vi "实验1-1.vi"() -> ()   [LabVIEW 2018]
panel:
  out "a*10":dbl
  out "?":bool
  in  "b":dbl
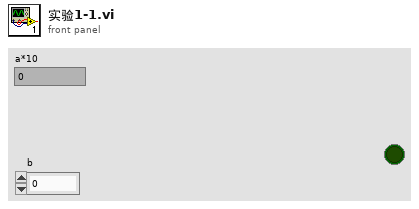
[diagram p1: front panel]
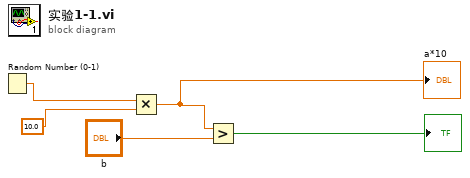
[diagram p0: block diagram]
diagram:
  n1 = Random Number (0-1)() -> (number: 0 to 1=w4:dbl)
  n2 = Multiply(x=w4, y=10.0) -> (x*y=w2:dbl)
  "a*10" <- w2
  n3 = Greater?(x=w2, y="b") -> (0:→"?":bool)
